vi "Set Int.vi"(8 "error in (no error)":errorcluster, 10 "Int":i32, 11 "IIntByVal in":refnum<class "IIntByVal.lvclass">) -> (0 "error out":errorcluster, 3 "IIntByVal out":refnum<class "IIntByVal.lvclass">)   [LabVIEW 2009, in "IIntByVal.lvclass"]
uses:
  IIntByVal.lvclass
  Numeric Test Object.lvclass
  Source/IUnknown Class/IUnknown.lvclass
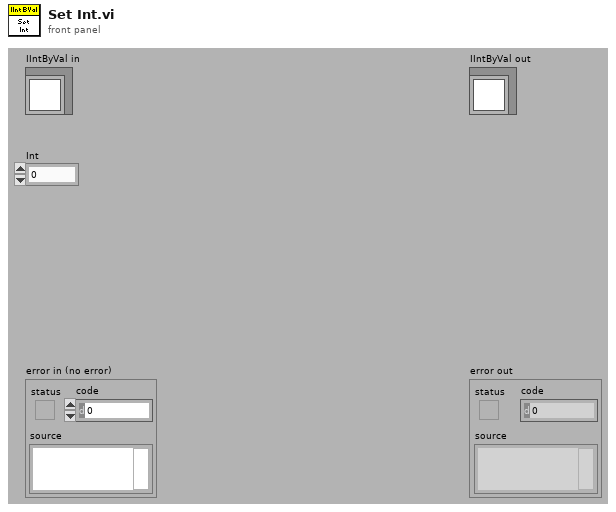
[diagram p1: front panel]
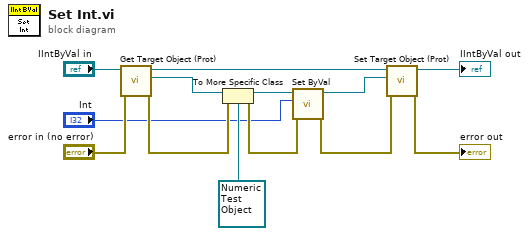
[diagram p0: block diagram]
diagram:
  n1 = call "Get Target Object (Prot).vi"("error in (no error)"="error in (no error)", "IUnknown in"="IIntByVal in") -> ("error out"=w10:errorcluster, "Target Object"=w9:refnum<class "Interfaceable.lvclass">, "IUnknown out"=w5:refnum<class "IIntByVal.lvclass">)  [unwired: 7 in]
  n2 = To More Specific Class(target class=refnum<class "Numeric Test Object.lvclass"> refnum ("Numeric.lvclass"), reference=w9, error in=w10) -> (specific class reference=w8:refnum<class "Numeric Test Object.lvclass">, error out=w7:errorcluster)
  n3 = call-dynamic "Set ByVal.vi"("error in (no error)"=w7, "Int"="Int", "Numeric in"=w8) -> ("error out"=w2:errorcluster, "Numeric out"=w3:refnum<class "Numeric Test Object.lvclass">)  [unwired: 7 in]
  n4 = call "Set Target Object (Prot).vi"("error in (no error)"=w2, "Target Object"=w3, "IUnknown in"=w5) -> ("error out"=→"error out":errorcluster, "IUnknown out"=→"IIntByVal out":refnum<class "IIntByVal.lvclass">)  [unwired: 7 in]
